vi "T2_KeyToValue_Fail.vi"(4 "Keys":cluster{"Start":u64, "End":u64}[](array[cluster]), 5 "String":string) -> (0 "Source > Dest":T1(c390), 1 "Values":cluster{"Start":u64, "End":u64}[](array[cluster]))   [LabVIEW 2022 SP3]
uses:
  f2448537-1bfe-4ed2-85b6-53f2f6bc46f2.vi
panel:
  out "Array 3":bool[](array[boolean])
  out "Array":u32[](array[numeric])
  out "appended array":bool[][](array[boolean])
  out "Array 2":cluster{"Start":u64, "End":u64}[][](array[cluster])
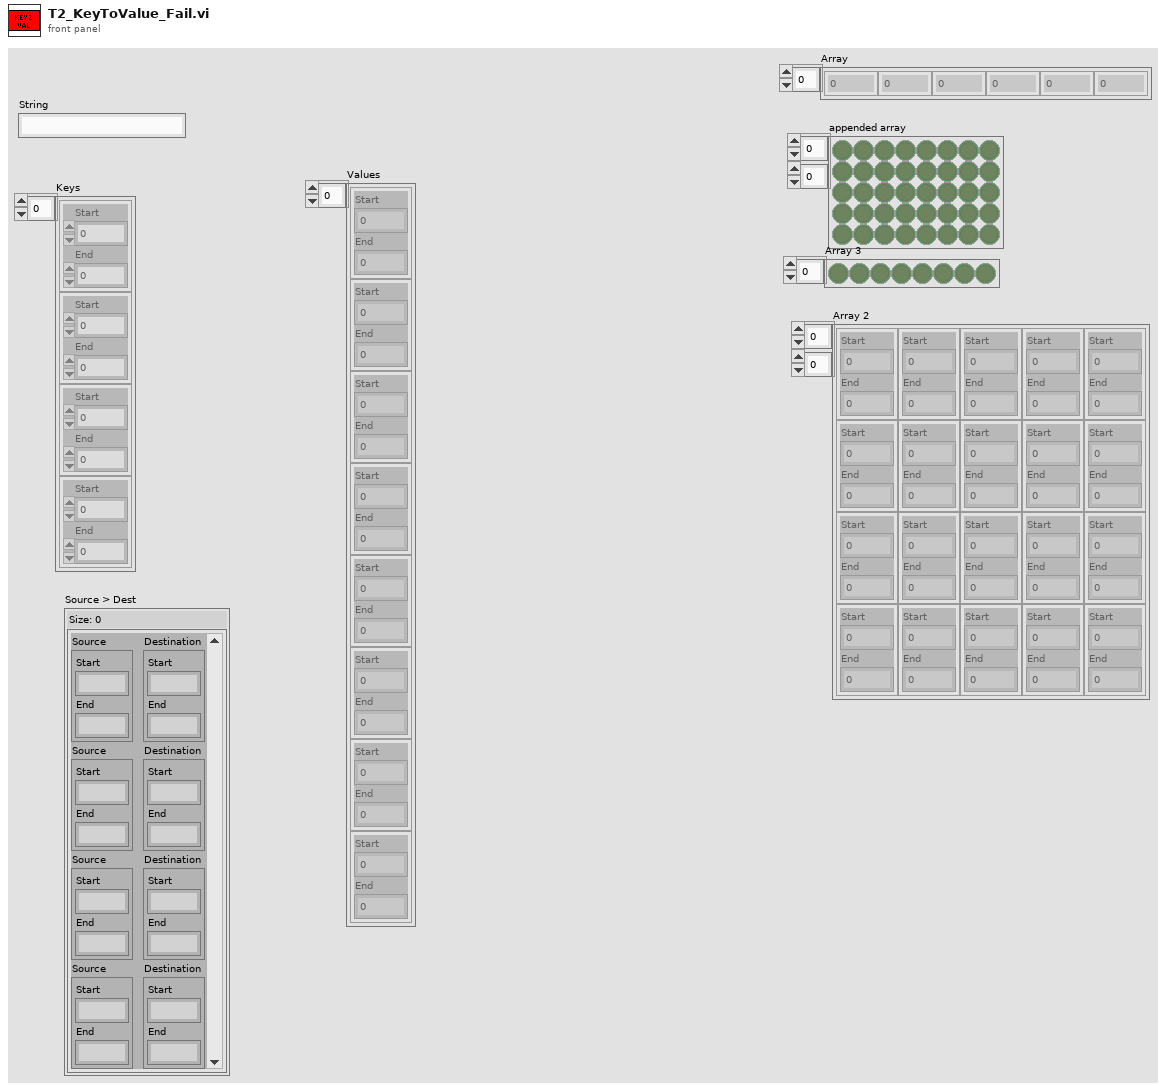
[diagram p1: front panel]
types:
  T1 = map{cluster{"Start":u64, "End":u64}, cluster{"Start":u64, "End":u64}}
  T2 = map{cluster{"Start":i64, "End":i64}, cluster{"Start":i64, "End":i64}}
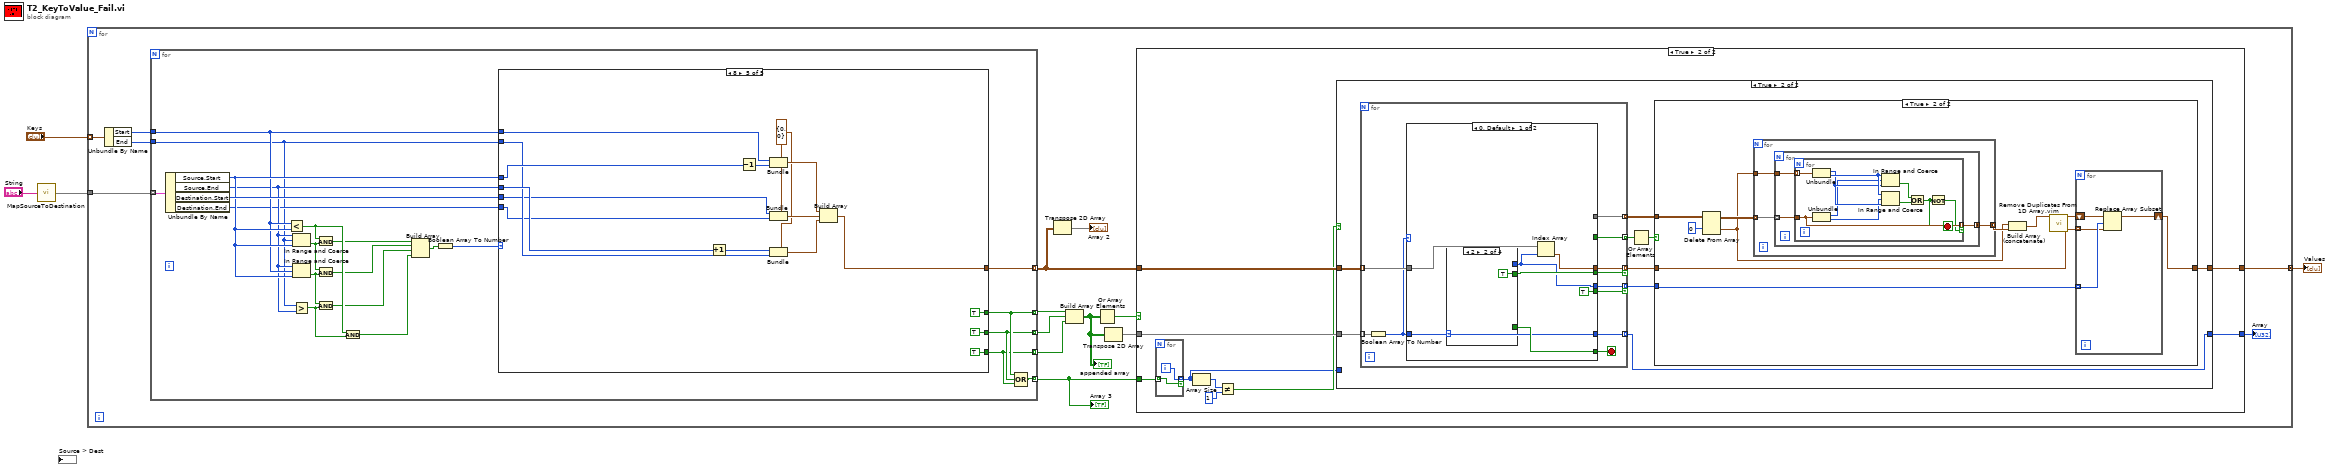
[diagram p0: block diagram]
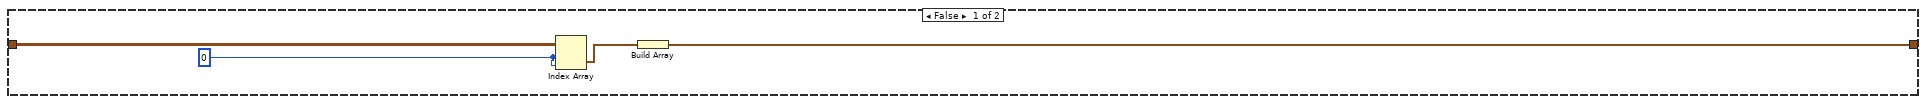
[diagram p2: hidden frame]
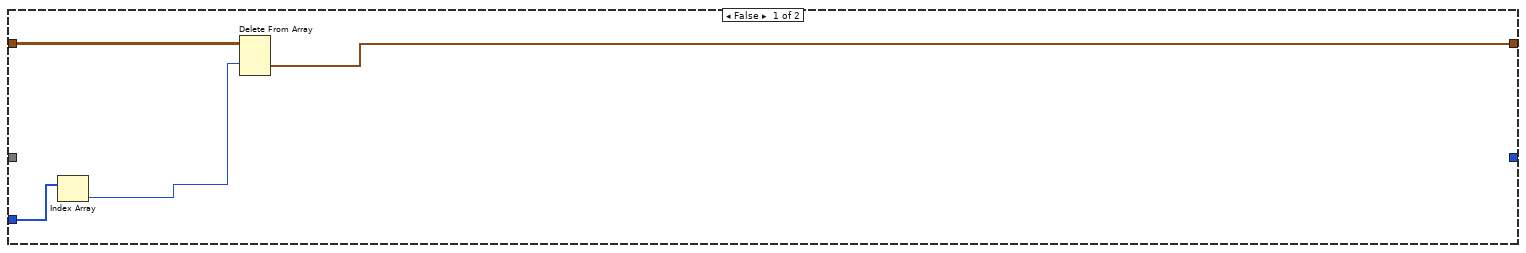
[diagram p3: hidden frame]
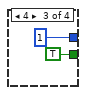
[diagram p6: hidden frame]
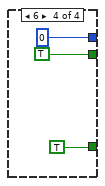
[diagram p7: hidden frame]
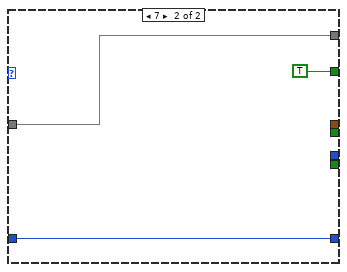
[diagram p8: hidden frame]
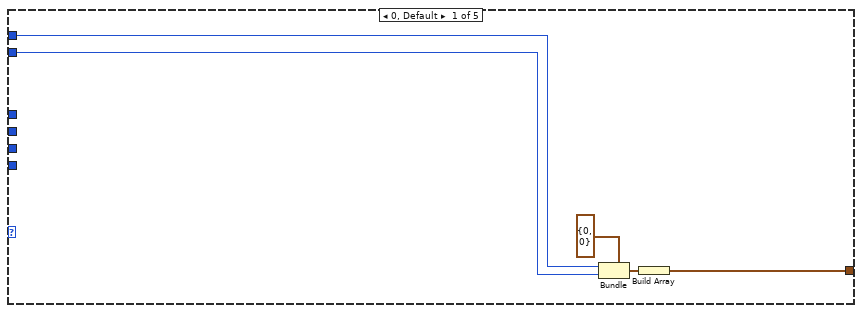
[diagram p9: hidden frame]
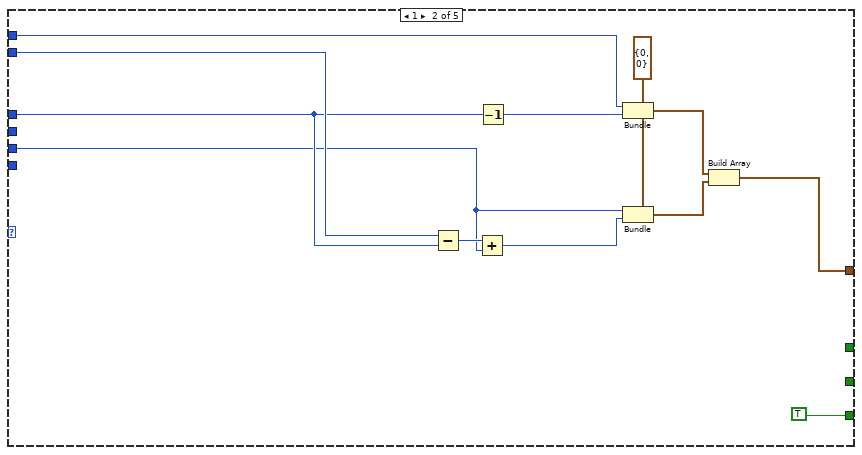
[diagram p10: hidden frame]
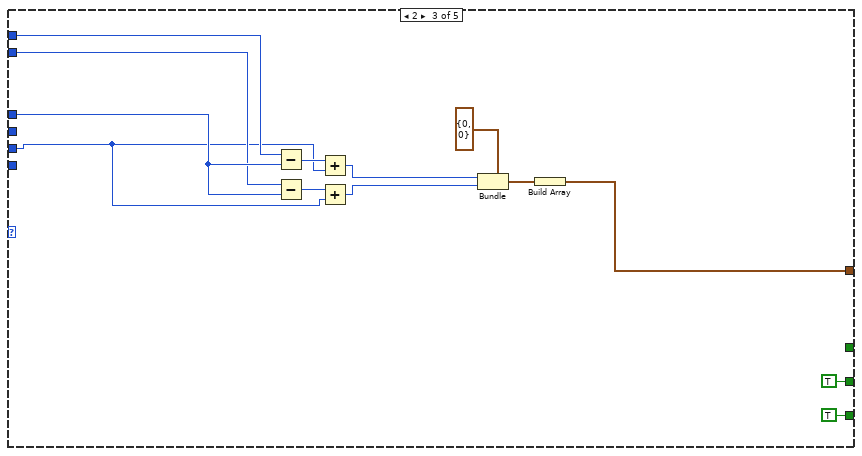
[diagram p11: hidden frame]
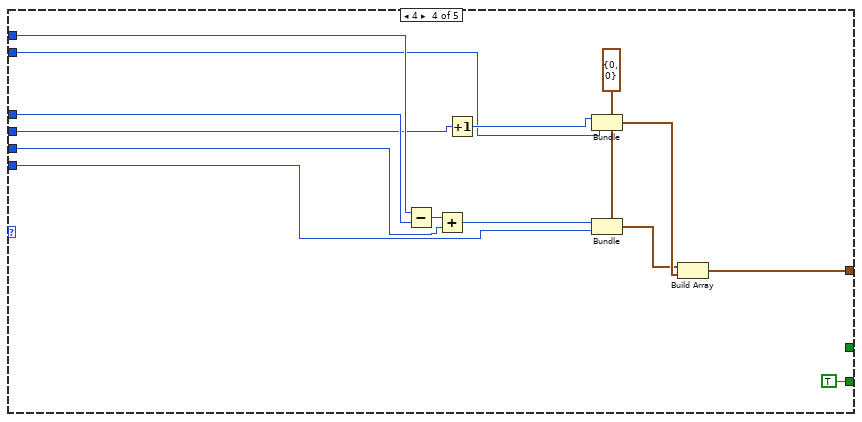
[diagram p12: hidden frame]
diagram:
  n1 = call "MapSourceToDestination.vi"("String"="String") -> ("Source > Dest"=w3:T2)  [unwired: 6 in]
  n2 = for {
    tunnel: "Keys" -> [w19] mode=indexing
    tunnel: w3 -> [w17]
    tunnel: [w9] -> w1 mode=concatenating
    n3 = Unbundle By Name(w19) -> ("Start"=w18:u64, "End"=w16:u64)
    n4 = for {
      tunnel: w17 -> [w127] mode=indexing
      tunnel: w18 -> [w124]
      tunnel: w16 -> [w111]
      tunnel: [w110] -> w10 mode=indexing
      tunnel: [w108] -> w14 mode=indexing
      tunnel: [w107] -> w13 mode=indexing
      tunnel: [w109] -> w15 mode=indexing
      tunnel: [w106] -> w5 mode=indexing
      n5 = Unbundle By Name(w127) -> ("Source.Start"=w125:i64, "Source.End"=w122:i64, "Destination.Start"=w126:i64, "Destination.End"=w112:i64)
      n6 = Less?(x=w124, y=w125) -> (x < y?=w120:bool)
      n7 = In Range and Coerce(upper limit=w122, x=w111, lower limit=w125) -> (In Range?=w123:bool)  [unwired: 1 out]
      n8 = In Range and Coerce(upper limit=w122, x=w124, lower limit=w125) -> (In Range?=w121:bool)  [unwired: 1 out]
      n9 = Greater?(x=w111, y=w122) -> (0:w119:bool)
      n10 = And(x=w120, y=w123) -> (x .and. y?=w118:bool)
      n11 = And(x=w123, y=w121) -> (x .and. y?=w117:bool)
      n12 = And(x=w121, y=w119) -> (x .and. y?=w116:bool)
      n13 = And(x=w120, y=w119) -> (x .and. y?=w115:bool)
      n14 = Build Array(w118, w117, w116, w115) -> (w114:bool[])
      n15 = Boolean Array To Number(Boolean array=w114) -> (number=w113:u32)
      n16 = case shown="8" w113 {
        tunnel: [w130 w144 w147 w159 w175] -> w110
        tunnel: w111 -> [w129 w136 w149 w160 w178]
        tunnel: w124 -> [w128 w137 w151 w167 w181]
        tunnel: w125 -> [_ w135 w150 w166 w180]
        tunnel: w122 -> [_ _ _ w162 w179]
        tunnel: w126 -> [_ w134 w148 w164 w177]
        tunnel: w112 -> [_ _ _ w163 w176]
        tunnel: [_ _ TRUE TRUE TRUE] -> w108
        tunnel: [_ TRUE TRUE _ TRUE] -> w107
        tunnel: [_ _ _ _ TRUE] -> w109
        frame 0, Default {
          n17 = Bundle(cluster=cluster{"Start":u64, "End":u64} {"Start"=0, "End"=0} ("Source"), "Start"=w128, "End"=w129) -> (w131:cluster{"Start":u64, "End":u64})
          n18 = Build Array(w131) -> (w130:cluster{"Start":u64, "End":u64}[])
        }
        frame 1 {
          w143 = cluster{"Start":u64, "End":u64} {"Start"=0, "End"=0} ("Source")
          n19 = Subtract(x=w136, y=w135) -> (x-y=w139:u64)
          n20 = Add(x=w139, y=w134) -> (x+y=w138:u64)
          n21 = Decrement(x=w135) -> (x-1=w142:i64)
          n22 = Bundle(cluster=w143, "Start"=w137, "End"=w142) -> (w141:cluster{"Start":u64, "End":u64})
          n23 = Bundle(cluster=w143, "Start"=w134, "End"=w138) -> (w140:cluster{"Start":u64, "End":u64})
          n24 = Build Array(w141, w140) -> (w144:cluster{"Start":u64, "End":u64}[])
        }
        frame 2 {
          n25 = Subtract(x=w151, y=w150) -> (x-y=w155:u64)
          n26 = Subtract(x=w149, y=w150) -> (x-y=w154:u64)
          n27 = Add(x=w155, y=w148) -> (x+y=w153:u64)
          n28 = Add(x=w154, y=w148) -> (x+y=w152:u64)
          n29 = Bundle(cluster=cluster{"Start":u64, "End":u64} {"Start"=0, "End"=0} ("Source"), "Start"=w153, "End"=w152) -> (w156:cluster{"Start":u64, "End":u64})
          n30 = Build Array(w156) -> (w147:cluster{"Start":u64, "End":u64}[])
        }
        frame 4 {
          w171 = cluster{"Start":u64, "End":u64} {"Start"=0, "End"=0} ("Source")
          n31 = Subtract(x=w167, y=w166) -> (x-y=w168:u64)
          n32 = Add(x=w168, y=w164) -> (x+y=w165:u64)
          n33 = Increment(x=w162) -> (x+1=w161:i64)
          n34 = Bundle(cluster=w171, "Start"=w161, "End"=w160) -> (w170:cluster{"Start":u64, "End":u64})
          n35 = Bundle(cluster=w171, "Start"=w165, "End"=w163) -> (w169:cluster{"Start":u64, "End":u64})
          n36 = Build Array(w169, w170) -> (w159:cluster{"Start":u64, "End":u64}[])
        }
        frame 8 {
          w184 = cluster{"Start":u64, "End":u64} {"Start"=0, "End"=0} ("Source")
          n37 = Increment(x=w179) -> (x+1=w182:i64)
          n38 = Decrement(x=w180) -> (x-1=w183:i64)
          n39 = Bundle(cluster=w184, "Start"=w181, "End"=w183) -> (w187:cluster{"Start":u64, "End":u64})
          n40 = Bundle(cluster=w184, "Start"=w177, "End"=w176) -> (w186:cluster{"Start":u64, "End":u64})
          n41 = Bundle(cluster=w184, "Start"=w182, "End"=w178) -> (w185:cluster{"Start":u64, "End":u64})
          n42 = Build Array(w187, w186, w185) -> (w175:cluster{"Start":u64, "End":u64}[])
        }
      }
      n43 = Compound Arithmetic op=OR(w109, w108, w107) -> (w106:bool)
    }
    "Array 3" <- w5
    n44 = Transpose 2D Array(2D array=w10) -> (transposed array=→"Array 2":cluster{"Start":u64, "End":u64}[][])
    n45 = Build Array(w15, w14, w13) -> (w8:bool[][])
    "appended array" <- w8
    n46 = Or Array Elements(Boolean array=w8) -> (logical OR=w11:bool)
    n47 = Transpose 2D Array(2D array=w8) -> (transposed array=w6:bool[][])
    n48 = case shown="True" w11 {
      tunnel: w10 -> [w23 w32]
      tunnel: [w20 w31] -> w9
      tunnel: w6 -> [_ w30]
      tunnel: [_ w29] -> w7
      tunnel: w5 -> [_ w28]
      frame False {
        w22 = 0 ("index (row)")
        n49 = Index Array(array=w23, index (row)=w22, index (col)=w22) -> (element=w21:cluster{"Start":u64, "End":u64})
        n50 = Build Array(w21) -> (w20:cluster{"Start":u64, "End":u64}[])
      }
      frame True {
        n51 = for {
          tunnel: w28 -> [w34] mode=indexing
          tunnel: [w33] -> w24 mode=indexing if=w34
          i -> [w33]
        }
        n52 = Array Size(array=w24) -> (size(s)=w26:i32)
        n53 = Not Equal?(x=w26, y=1) -> (x != y?=w25:bool)
        n54 = case shown="True" w25 {
          tunnel: w32 -> [w38 w47]
          tunnel: [w37 w43] -> w31
          tunnel: w30 -> [_ w46]
          tunnel: [_ w39] -> w29
          tunnel: w24 -> [w35 _]
          frame False {
            n55 = Index Array(array=w35) -> (element=w36:i32)  [unwired: 1 in]
            n56 = Delete From Array(array=w38, index (row)=w36) -> (deleted portion=w37:cluster{"Start":u64, "End":u64}[])  [unwired: 2 in, 1 out]
          }
          frame True {
            n57 = for {
              tunnel: w47 -> [w86] mode=indexing
              tunnel: [w87] -> w42 mode=indexing if=w88
              tunnel: w46 -> [w85] mode=indexing
              tunnel: [w83] -> w40 mode=indexing if=w82
              tunnel: [w81] -> w41 mode=indexing
              tunnel: [w80] -> w45 mode=indexing
              tunnel: [w79] -> w39 mode=indexing
              stop <- w89 stop-if-true
              n58 = Boolean Array To Number(Boolean array=w85) -> (number=w84:u32)
              n59 = case shown="0, Default" w84 {
                tunnel: [w93 _] -> w89
                tunnel: [w96 _] -> w88
                tunnel: [w95 _] -> w87
                tunnel: w86 -> [w94 w105]
                tunnel: w84 -> [w90 w103]
                tunnel: [w91 _] -> w83
                tunnel: [TRUE _] -> w82
                tunnel: [_ w105] -> w81
                tunnel: [_ TRUE] -> w80
                tunnel: [w90 w103] -> w79
                frame 0, Default {
                  n60 = case shown="2" w90 {
                    tunnel: [_ _ _ TRUE] -> w93
                    tunnel: [_ TRUE TRUE TRUE] -> w96
                    tunnel: [_ _ 1 0 ("index")] -> w91
                    frame 0, Default {
                    }
                    frame 2 {
                    }
                    frame 4 {
                    }
                    frame 6 {
                    }
                  }
                  n61 = Index Array(array=w94, index=w91) -> (element=w95:cluster{"Start":u64, "End":u64})
                }
                frame 7 {
                }
              }
            }
            n62 = Or Array Elements(Boolean array=w45) -> (logical OR=w44:bool)
            n63 = case shown="True" w44 {
              tunnel: [w48 w56] -> w43
              tunnel: w42 -> [w48 w57]
              tunnel: w41 -> [_ w55]
              tunnel: w40 -> [_ w58]
              frame False {
              }
              frame True {
                n64 = Delete From Array(array=w55, index (row)=0) -> (deleted portion=w51:cluster{"Start":u64, "End":u64}[], array with subset deleted=w53:cluster{"Start":u64, "End":u64}[][])  [unwired: 2 in]
                n65 = for {
                  tunnel: w51 -> [w60]
                  tunnel: w53 -> [w61] mode=indexing
                  tunnel: [w59] -> w52 mode=concatenating
                  n66 = for {
                    tunnel: w61 -> [w63] mode=indexing
                    tunnel: w60 -> [w64]
                    tunnel: [w62] -> w59 mode=concatenating
                    n67 = for {
                      tunnel: w64 -> [w74] mode=indexing
                      tunnel: w63 -> [w67]
                      tunnel: [w67] -> w62 mode=indexing if=w66
                      stop <- w65 stop-if-true
                      n68 = Unbundle(w74) -> ("Start"=w72:u64, "End"=w73:u64)
                      n69 = Unbundle(w67) -> ("Start"=w71:u64, "End"=w70:u64)
                      n70 = In Range and Coerce(upper limit=w73, x=w71, lower limit=w72) -> (In Range?=w69:bool)  [unwired: 1 out]
                      n71 = In Range and Coerce(upper limit=w73, x=w70, lower limit=w72) -> (In Range?=w68:bool)  [unwired: 1 out]
                      n72 = Or(x=w69, y=w68) -> (x .or. y?=w65:bool)
                      n73 = Not(x=w65) -> (.not. x?=w66:bool)
                    }
                  }
                }
                n74 = Build Array (concatenate)(w51, w52) -> (w50:cluster{"Start":u64, "End":u64}[])
                n75 = call "Remove Duplicates From 1D Array.vim"("array"=w50) -> ("array with duplicates removed"=w49:cluster{"Start":u64, "End":u64}[])  [unwired: 10 in]
                n76 = for {
                  shift-right: [w77] -> w56
                  shift-left: w49 -> [w78]
                  tunnel: w58 -> [w76] mode=indexing
                  tunnel: w57 -> [w75] mode=indexing
                  n77 = Replace Array Subset(array=w78, new element=w75, index=w76) -> (w77:cluster{"Start":u64, "End":u64}[])
                }
              }
            }
          }
        }
      }
    }
    "Array" <- w7
  }
  "Values" <- w1
